vi "Calculate TimerDRV Period.vi"(8 "error in (no error)":errorcluster, 11 "TimerDRV in":refnum<class "TimerDRV.lvclass">) -> (0 "error out":errorcluster, 3 "TimerDRV out":refnum<class "TimerDRV.lvclass">)   [LabVIEW 2019, in "TimingDRV Engine.lvlib" / "TimerDRV.lvclass"]
uses:
  TimerDRV.lvclass
  TimerDRV.lvclass/TimerDRV.ctl
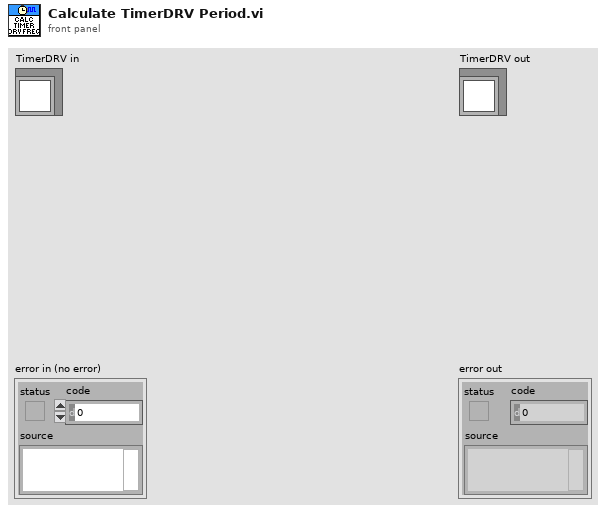
[diagram p1: front panel]
types:
  T1 = typedef "TimingDRV Engine.lvlib/TimerDRV.lvclass/Target Type.ctl" = enum16{"PharLap", "VxWorks", "Windows", "Linux_32_ARM", "Linux_x64"}
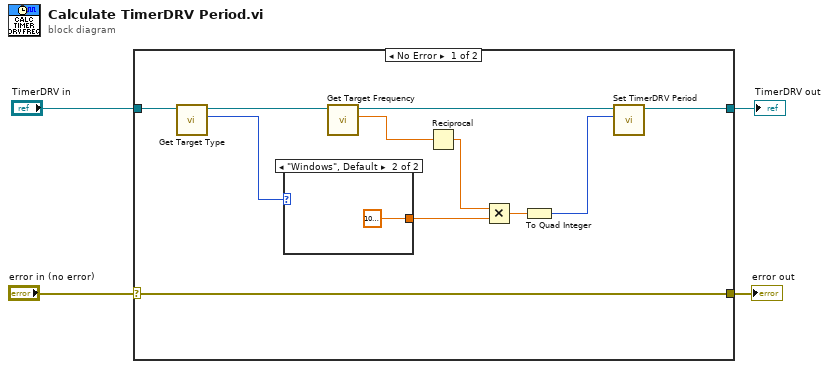
[diagram p0: block diagram]
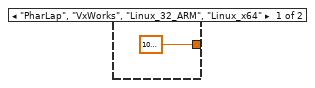
[diagram p2: hidden frame]
diagram:
  n1 = case shown="No Error" "error in (no error)" {
    selector: "error in (no error)" -> [w5 w19]
    tunnel: [w5 w19] -> w3
    tunnel: [w9 w18] -> w1
    tunnel: "TimerDRV in" -> [w14 w18]
    frame No Error {
      n2 = call "Get Target Type.vi"("TimerDRV in"=w14) -> ("Target Type"=w6:T1, "TimerDRV out"=w12:refnum<class "TimerDRV.lvclass">)  [unwired: 9 in]
      n3 = case shown="\"Windows\", Default" w6 {
        tunnel: [1000000.0 ("Target Frequency") 1000.0 ("Target Frequency")] -> w7
        frame "PharLap", "VxWorks", "Linux_32_ARM", "Linux_x64" {
        }
        frame "Windows", Default {
        }
      }
      n4 = call "Get Target Frequency.vi"("TimerDRV in"=w12) -> ("Target Frequency"=w15:dbl, "TimerDRV out"=w10:refnum<class "TimerDRV.lvclass">)  [unwired: 9 in]
      n5 = Reciprocal(x=w15) -> (1/x=w13:dbl)
      n6 = Multiply(x=w13, y=w7) -> (x*y=w11:dbl)
      n7 = To Quad Integer(1:w11) -> (0:w8:i64)
      n8 = call "Set TimerDRV Period.vi"("TimerDRV Period"=w8, "TimerDRV in"=w10) -> ("TimerDRV out"=w9:refnum<class "TimerDRV.lvclass">)  [unwired: 9 in]
    }
    frame Error {
    }
  }
  "error out" <- w3
  "TimerDRV out" <- w1
